vi "monitorFileSize.vi"(8 "error in (no error)":errorcluster, 11 "Logger in":refnum<class "Log.lvclass">) -> (0 "error out":errorcluster, 1 "newValue?":bool, 2 "logFilePath":path, 3 "Logger out":refnum<class "Log.lvclass">)   [LabVIEW 2013, in "Log.lvclass"]
uses:
  Log.lvclass
  Log.lvclass/Log.ctl
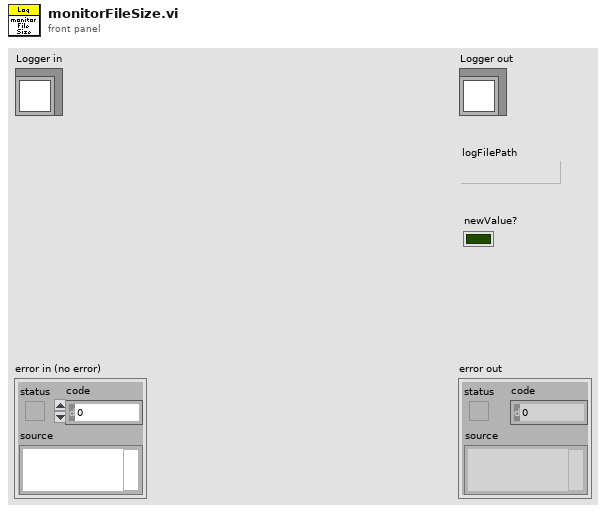
[diagram p1: front panel]
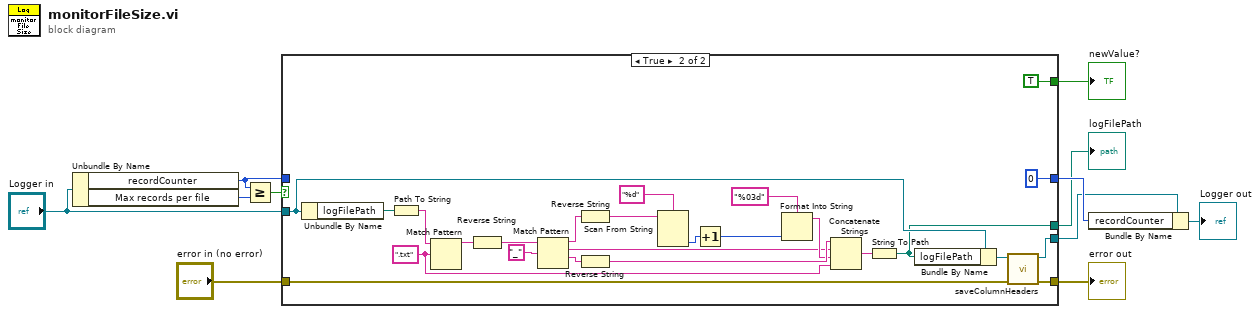
[diagram p0: block diagram]
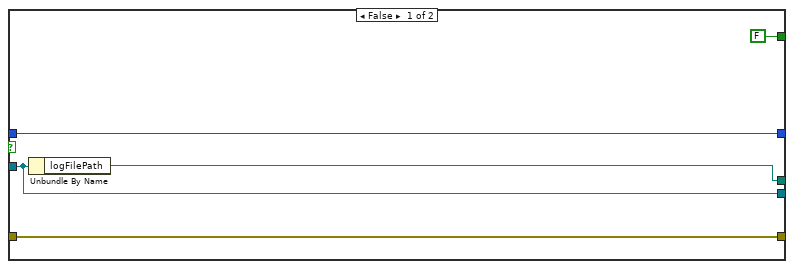
[diagram p2: hidden frame]
diagram:
  n1 = Unbundle By Name("Logger in") -> ("recordCounter"=w3:u32, "Max records per file"=w9:u32)
  n2 = Greater Or Equal?(x=w3, y=w9) -> (x >= y?=w8:bool)
  n3 = case shown="True" w8 {
    tunnel: w3 -> [w15 _]
    tunnel: [w15 u32 0] -> w11
    tunnel: "Logger in" -> [w14 w28]
    tunnel: [w14 w21] -> w10
    tunnel: [w16 w20] -> w5
    tunnel: "error in (no error)" -> [w16 w19]
    tunnel: [w13 w18] -> w2
    tunnel: [FALSE TRUE] -> w1
    frame False {
      n4 = Unbundle By Name(w14) -> ("logFilePath"=w13:path)
    }
    frame True {
      w29 = ".txt" ("regular expression")
      n5 = Unbundle By Name(w28) -> ("logFilePath"=w27:path)
      n6 = Path To String(path=w27) -> (string=w40:string)
      n7 = Match Pattern(string=w40, regular expression=w29) -> (before substring=w39:string)  [unwired: 1 in, 3 out]
      n8 = Reverse String(1:w39) -> (0:w38:string)
      n9 = Match Pattern(string=w38, regular expression="_") -> (before substring=w35:string, match substring=w24:string, after substring=w33:string)  [unwired: 1 in, 1 out]
      n10 = Reverse String(1:w35) -> (0:w23:string)
      n11 = Reverse String(1:w33) -> (0:w31:string)
      n12 = Scan From String(format string="%d", input string=w23) -> (output 1=w34:i32)  [unwired: 3 in, 3 out]
      n13 = Increment(x=w34) -> (x+1=w32:i32)
      n14 = Format Into String(format string="%03d", w32) -> (resulting string=w30:string)  [unwired: 2 in, 1 out]
      n15 = Concatenate Strings(w31, w24, w30, w29) -> (w26:string)
      n16 = String To Path(string=w26) -> (path=w18:path)
      n17 = Bundle By Name(cluster=w28, "logFilePath"=w18) -> (w22:refnum<class "Log.lvclass">)
      n18 = call "saveColumnHeaders.vi"("error in (no error)"=w19, "Logger in"=w22) -> ("error out"=w20:errorcluster, "Logger out"=w21:refnum<class "Log.lvclass">)  [unwired: 8 in]
    }
  }
  "error out" <- w5
  "logFilePath" <- w2
  "newValue?" <- w1
  n19 = Bundle By Name(cluster=w10, "recordCounter"=w11) -> (→"Logger out":refnum<class "Log.lvclass">)
